vi "Handle Zoom Event.vi"(6 "Coords":T1, 8 "error in":errorcluster, 9 "Zoom History":cluster{"X":sgl, "Y":sgl}[](array[cluster]), 10 "Zoom Type":enum32{"Zoom In", "Zoom Out"}(ring)=enum."Zoom Out", 11 "BigMAQ in":refnum<class "BigMAQ.lvclass">) -> (0 "error out":errorcluster, 1 "Discard?":bool, 2 "Zoom Out?":bool, 3 "BigMAQ out":refnum<class "BigMAQ.lvclass">)   [LabVIEW 2019, in "BigMAQ.lvclass"]
uses:
  BigMAQ.lvclass
  <vilib>/Utility/miscctls.llb/LVPoint32TypeDef.ctl
  BigMAQ.lvclass/BigMAQ.ctl
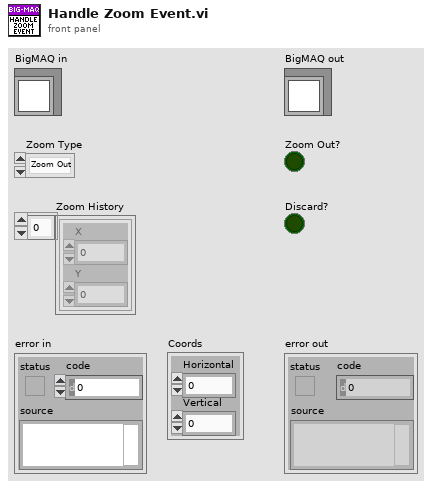
[diagram p1: front panel]
types:
  T1 = typedef "LVPoint32TypeDef.ctl" = cluster{"Horizontal":i32, "Vertical":i32}
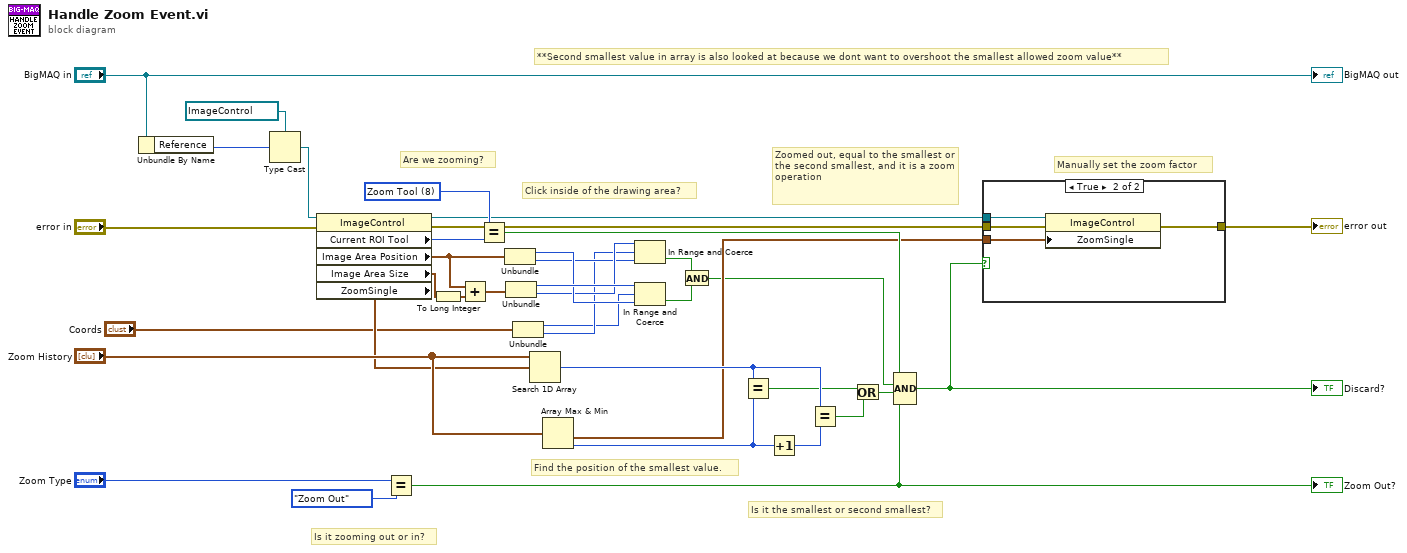
[diagram p0: block diagram]
diagram:
  w37 = u32 8 items=["Zoom Tool"=8, "Selection Tool"=0, "Pan Tool"=9, "Point Tool"=1, "Line Tool"=2, "Rectangle Tool"=3, "Rotated Rectangle Tool"=12, "Polyline Tool"=10, "Polygon Tool"=5, "Freehand Tool"=11, "Closed Freehand Tool"=6, "Ellipse Tool"=4, "Annulus Tool"=7] ("Current ROI Tool")
  # "Manually set the zoom factor"
  # "Are we zooming?"
  # "**Second smallest value in array is also looked at because we dont want to overshoot the smallest allowed zoom value**"
  # "Is it the smallest or second smallest?"
  # "Find the position of the smallest value."
  # "Is it zooming out or in?"
  # "Click inside of the drawing area?"
  # "Zoomed out, equal to the smallest or the second smallest, and it is a zoom operation"
  n1 = Unbundle By Name("BigMAQ in") -> ("Reference"=w34:i32)
  n2 = Type Cast(type=refnum<vi> refnum ("reference"), x=w34) -> (*(type *) &x=w16:refnum<vi>)
  n3 = property class="ImageControl"(reference=w16, error in="error in") -> (reference out=w23:refnum<vi>, error out=w20:errorcluster, "Current ROI Tool"=w36:u32, "Image Area Position"=w12:cluster{"Left":i32, "Top":i32}, "Image Area Size"=w15:cluster{"Width":u32, "Height":u32}, "ZoomSingle"=w14:cluster{"X":sgl, "Y":sgl})
  n4 = Equal?(x="Zoom Type", y=enum32{"Zoom In", "Zoom Out"}."Zoom Out" ("Zoom Type")) -> (x = y?=w27:bool)
  "Zoom Out?" <- w27
  n5 = To Long Integer(number=w15) -> (32bit integer=w3:cluster{"Width":i32, "Height":i32})
  n6 = Add(x=w12, y=w3) -> (x+y=w13:cluster{i32, i32})
  n7 = Equal?(x=w37, y=w36) -> (x = y?=w25:bool)
  n8 = Unbundle(w12) -> ("Left"=w10:i32, "Top"=w8:i32)
  n9 = Unbundle(w13) -> (w11:i32, w9:i32)
  n10 = Unbundle("Coords") -> ("Horizontal"=w2:i32, "Vertical"=w6:i32)
  n11 = Search 1D Array(1D array="Zoom History", element=w14) -> (index of element=w29:i32)  [unwired: 1 in]
  n12 = Array Max & Min(array="Zoom History") -> (min value=w22:cluster{"X":sgl, "Y":sgl}, min index (indices)=w31:i32)  [unwired: 2 out]
  n13 = In Range and Coerce(upper limit=w9, x=w6, lower limit=w8) -> (In Range?=w5:bool)  [unwired: 1 out]
  n14 = In Range and Coerce(upper limit=w11, x=w2, lower limit=w10) -> (In Range?=w4:bool)  [unwired: 1 out]
  n15 = And(x=w5, y=w4) -> (x .and. y?=w1:bool)
  n16 = Equal?(x=w29, y=w31) -> (x = y?=w28:bool)
  n17 = Increment(x=w31) -> (x+1=w30:i32)
  n18 = Equal?(x=w29, y=w30) -> (x = y?=w21:bool)
  n19 = Or(x=w28, y=w21) -> (x .or. y?=w26:bool)
  n20 = Compound Arithmetic op=AND(w25, w1, w26, w27) -> (w24:bool)
  "Discard?" <- w24
  n21 = case shown="True" w24 {
    tunnel: w23 -> [_ w43]
    tunnel: w22 -> [_ w42]
    tunnel: [w39 w41] -> w18
    tunnel: w20 -> [w39 w40]
    frame False {
    }
    frame True {
      n22 = property class="ImageControl"(reference=w43, error in=w40, "ZoomSingle"=w42) -> (error out=w41:errorcluster)  [unwired: 1 out]
    }
  }
  "error out" <- w18
  "BigMAQ out" <- "BigMAQ in"
